vi "Robot Global Data.vi"() -> ()   [LabVIEW 2014]
doc: "This global VI can contain as many global variables as you need. Place a control on the panel, give it a good name. To read or write to it from a VI, drag the icon to the diagram of that VI. You can also drag from the project. Click on the node to change which global you access. You shouldn't have multiple locations writing to a global or it will cause a race-condition."
uses:
  <vilib>/Rock Robotics/WPI/Camera/WPI_CameraImageSize.ctl
  <vilib>/Rock Robotics/WPI/DriverStation/WPI_DriverStationRobotMode2.ctl
  Vector.ctl
  DriveControl.ctl
  TeleopDriveGroup.ctl
panel:
  out "Safety Override":bool
  out "Lift Mode Override":bool
  out "Auto-DeLooper":bool
  out "CanGrab":bool
  out "CanStable":bool
  out "AutoDriveReached":bool
  out "Time":dbl
  in  "Lift Setpoint M":dbl
  in  "Lift Movement":dbl
  in  "TeleopDrive":T1
  in  "ManagerRobotMode":enum16{"Autonomous", "Disabled", "Teleop"}(ring)
  out "IntakeShouldAcuate":bool
  out "IsLiftZeroing":bool
  in  "Intake":dbl
  out "Intake Piston":bool
  in  "DriveMode":T2
  out "DisableIntakeManager":bool
  in  "Drive Vector":T3
  in  "IntakeMultiplier":dbl
  out "DisableTalonManager":bool
  out "DisablePnumaticsControl":bool
  out "DisableRumbleManager":bool
  out "DriveReachedSetpoint":bool
  out "DisableDriveManager":bool
  out "Right Reached":bool
  out "Left Reached":bool
  in  "Tote Constant":dbl
  in  "Rumble Duration":dbl
  out "Brake Mode?":bool
  out "DisableLiftManager":bool
  out "Lift Zeroed":bool
  out "Grabber Zeroed":bool
  in  "Grabber Setpoint":dbl
  in  "MLP Report":T4 {"Orientation" format="%.2f"; "Dimensions"."Height" format="%.2f"; "Dimensions"."Width" format="%.2f"; "Center of Mass"."Y" format="%.2f"; "Center of Mass"."X" format="%.2f"; "Bounding Rect"."Bottom" format="%.2f"; "Bounding Rect"."Right" format="%.2f"; "Bounding Rect"."Top" format="%.2f"; "Bounding Rect"."Left" format="%.2f"; "Number of Holes" format="%.2f"; "Area" format="%.2f"}
  in  "Lift Setpoint":dbl
  out "Drive Shift":bool
  in  "Robot Mode":T5
  in  "image size":T6=enum."320x240"
  in  "Enable Vision":bool
  # "Base Robot Globals"
  # "Zeroed Indicators"
  # "Pnumatic Control Indicators"
  # "Manager Indicators"
  # "Lift Hard Setpoints"
  # "Indicators for disabling managers"
  # "Report for the Vision Particle"
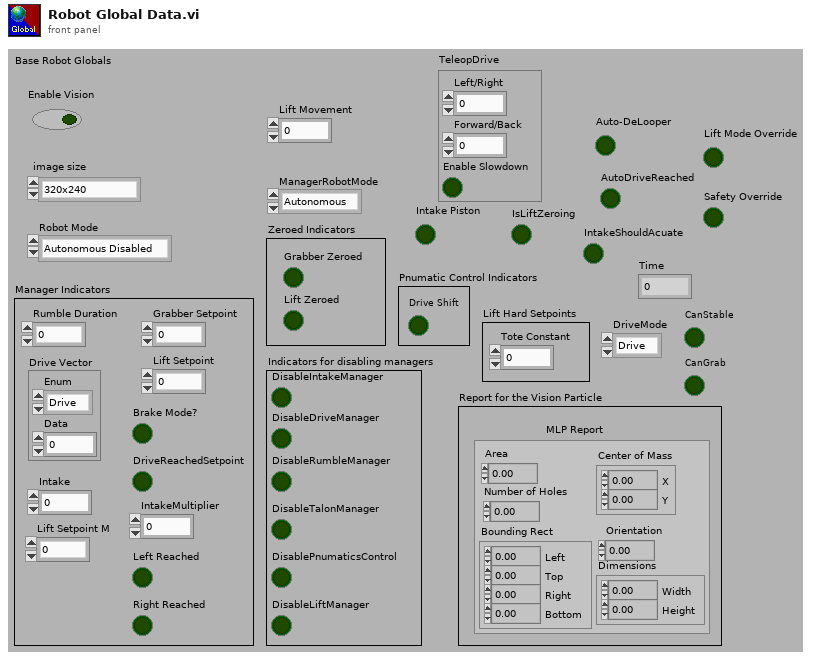
[diagram p1: front panel]
types:
  T1 = typedef "TeleopDriveGroup.ctl" = cluster{"Left/Right":dbl, "Forward/Back":dbl, "Enable Slowdown":bool}
  T2 = typedef "DriveControl.ctl" = enum16{"Drive", "Turn"}
  T3 = typedef "Vector.ctl" = cluster{"Enum":T2, "Data":dbl}
  T4 = cluster{"Area":dbl, "Number of Holes":dbl, "Bounding Rect":cluster{"Left":dbl, "Top":dbl, "Right":dbl, "Bottom":dbl}, "Center of Mass":cluster{"X":dbl, "Y":dbl}, "Orientation":dbl, "Dimensions":cluster{"Width":dbl, "Height":dbl}}
  T5 = typedef "WPI_DriverStationRobotMode2.ctl" = enum16{"Autonomous Disabled", "Autonomous Enabled", "Teleop Disabled", "Teleop Enabled", "Disconnected", "Finish", "Test Disabled", "Test Enabled", "Emergency Stopped"}
  T6 = typedef "WPI_CameraImageSize.ctl" = enum16{"640x480", "320x240", "160x120", "Custom"}
diagram:
